vi "From String Array.vi"(8 "error in (no error)":errorcluster, 9 "String Array":string[](array[string]), 11 "Update Tag Config in":refnum<class "Update Tag Config.lvclass">) -> (0 "error out":errorcluster, 1 "String Array 2":string[](array[string]), 3 "Update Tag Config out":refnum<class "Update Tag Config.lvclass">)   [LabVIEW 2015, in "Update Tag Config.lvclass"]
uses:
  Update Tag Config.lvclass
  <vilib>/NI/Tag Bus Module Framework/channel/channel classification.ctl
  <vilib>/NI/Tag Bus/tag/Data Type.ctl
  classes/Step/Config/Step Config.lvclass
  <vilib>/NI/Tag Bus Module Framework/channel/TBM channel.lvclass
  <vilib>/NI/Tag Bus/tag/tag descriptor.lvclass
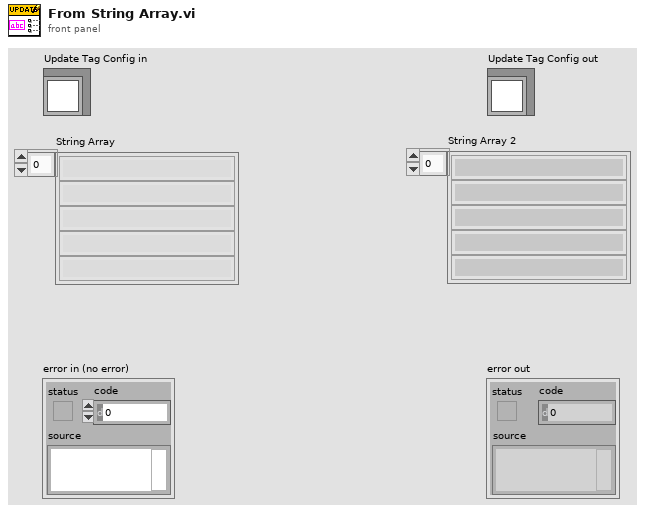
[diagram p1: front panel]
types:
  T1 = typedef "TBM channel.lvclass/channel classification.ctl" = enum16{"input data", "output data", "processing parameter", "processing result"}
  T2 = typedef "tag bus.lvlib/tag descriptor.lvclass/Data Type.ctl" = enum16{"Double", "Single", "I64", "I32", "I16", "I8", "U64", "U32", "U16", "U8", "Boolean", "String", "Array of Double", "Array of Single", "Array of I64", "Array of I32", "Array of I16", "Array of I8", "Array of U64", "Array of U32", "Array of U16", "Array of U8", "Array of Boolean", "Array of String"}
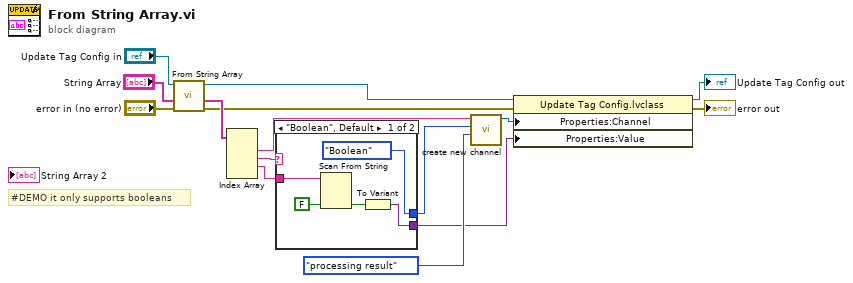
[diagram p0: block diagram]
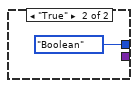
[diagram p2: hidden frame]
diagram:
  # "#DEMO it only supports booleans"
  n1 = call-parent "From String Array.vi"("error in (no error)"="error in (no error)", "String Array"="String Array", "Step Config in"="Update Tag Config in") -> ("error out"=w1:errorcluster, "Elements Left 2"=w5:string[], "Step Config out"=w4:refnum<class "Update Tag Config.lvclass">)  [unwired: 6 in]
  n2 = Index Array(array=w5) -> (element #1=w13:string, element #2=w12:string, element #3=w7:string)  [unwired: 4 in, 1 out]
  n3 = case shown="\"Boolean\", Default" w12 {
    tunnel: [Data_Type."Boolean" ("data type") Data_Type."Boolean" ("data type")] -> w11
    tunnel: [w17 _] -> w8
    tunnel: w7 -> [w16 _]
    frame "Boolean", Default {
      n4 = Scan From String(input string=w16, default 1=FALSE) -> (output 1=w18:bool)  [unwired: 3 in, 3 out]
      n5 = To Variant(anything=w18) -> (Variant=w17:variant)
    }
    frame "True" {
    }
  }
  n6 = call <vilib>:"create new channel.vi"("channel classification"=channel_classification."processing result", "data type"=w11, "channel name"=w13) -> ("channel"=w10:refnum<class "TBM channel.lvclass">)  [unwired: 8 in]
  n7 = property class="Update Tag Config.lvclass"(reference=w4, error in=w1, "Properties:Channel"=w10, "Properties:Value"=w8) -> (reference out=→"Update Tag Config out":refnum<class "Update Tag Config.lvclass">, error out=→"error out":errorcluster)
